vi "Parse Expression.vi"(11 "Expression":string) -> (0 "error out":errorcluster, 2 "Parsed Expression":T1)   [LabVIEW 2012]
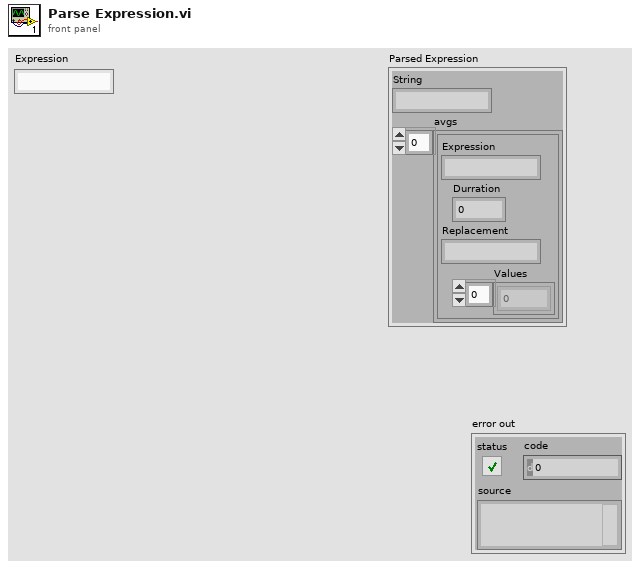
[diagram p1: front panel]
types:
  T1 = cluster{"String":string, "avgs":cluster{"Expression":string, "Durration":dbl, "Replacement":string, "Values":dbl[]}[]}
  T2 = cluster{"Expression":string, "Durration":dbl, "Replacement":string, "Values":dbl[]}[]
  T3 = cluster{"Expression":string, "Durration":dbl, "Replacement":string, "Values":dbl[]}
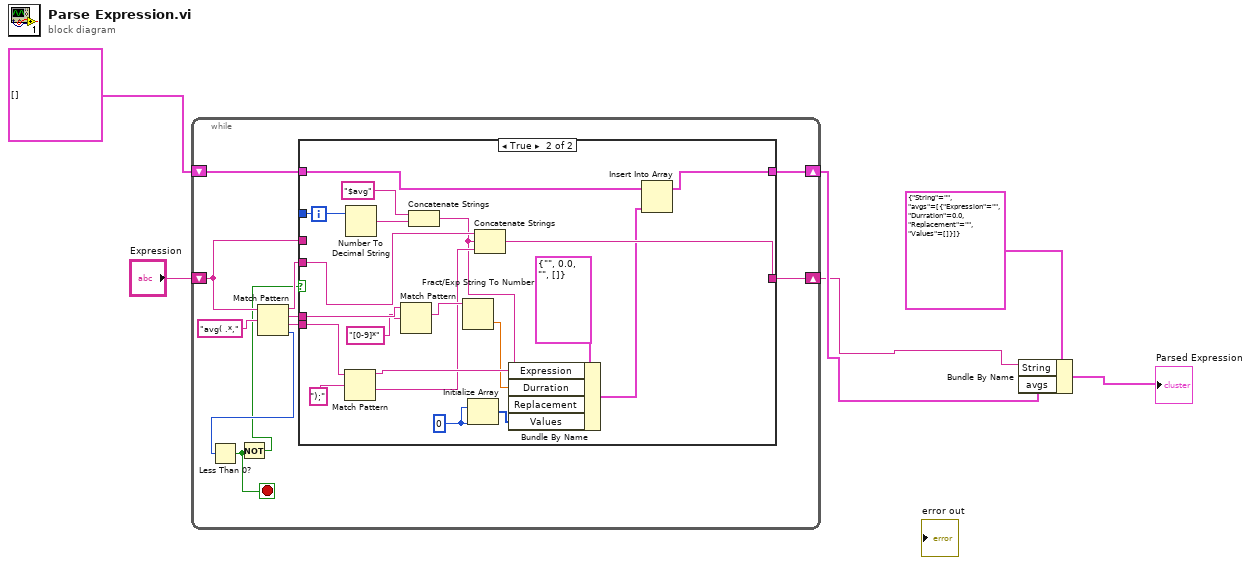
[diagram p0: block diagram]
diagram:
  n1 = while {
    shift-right: [w13] -> w1
    shift-left: "Expression" -> [w11]
    shift-right: [w7] -> w3
    shift-left: T2 [] -> [w8]
    i -> [w14]
    stop <- w9 stop-if-true
    n2 = Match Pattern(string=w11, regular expression="avg( .*,") -> (before substring=w15:string, match substring=w17:string, after substring=w16:string, offset past match=w12:i32)  [unwired: 1 in]
    n3 = Less Than 0?(x=w12) -> (x < 0?=w9:bool)
    n4 = Not(x=w9) -> (.not. x?=w10:bool)
    n5 = case shown="True" w10 {
      tunnel: w17 -> [_ w40]
      tunnel: w16 -> [_ w37]
      tunnel: w15 -> [_ w32]
      tunnel: w14 -> [_ w31]
      tunnel: [w20 w28] -> w13
      tunnel: w11 -> [w20 _]
      tunnel: w8 -> [w19 w23]
      tunnel: [w19 w22] -> w7
      frame False {
      }
      frame True {
        w25 = 0
        n6 = Match Pattern(string=w37, regular expression=");") -> (before substring=w36:string, after substring=w33:string)  [unwired: 1 in, 2 out]
        n7 = Number To Decimal String(number=w31) -> (decimal integer string=w30:string)  [unwired: 1 in]
        n8 = Match Pattern(string=w40, regular expression="[0-9]*") -> (match substring=w35:string)  [unwired: 1 in, 3 out]
        n9 = Concatenate Strings("$avg", w30) -> (w27:string)
        n10 = Fract/Exp String To Number(string=w35) -> (number=w34:dbl)  [unwired: 3 in, 1 out]
        n11 = Initialize Array(w25, w25) -> (w24:i32[])
        n12 = Concatenate Strings(w32, w27, w33) -> (w28:string)
        n13 = Bundle By Name(cluster=T3 {"Expression"="", "Durration"=0.0, "Replacement"="", "Values"=[]} ("Cluster"), "Expression"=w36, "Durration"=w34, "Replacement"=w27, "Values"=w24) -> (w21:T3)
        n14 = Insert Into Array(array=w23, new element=w21) -> (w22:T2)  [unwired: 1 in]
      }
    }
  }
  n15 = Bundle By Name(cluster=T1 {"String"="", "avgs"=[{"Expression"="", "Durration"=0.0, "Replacement"="", "Values"=[]}]} ("Expression"), "String"=w1, "avgs"=w3) -> (→"Parsed Expression":T1)
